vi "GPS -Nearest Points to Lat Lng.vi"(5 "Inputs":T1={" # Pts"=5, "PinDropLatDblClck"=0.0, "PinDropLngDblClck"=0.0, "AddrLat"=0.0, "AddrLng"=0.0, "tbVw"=enum."Position"}, 11 "error in (no error)":errorcluster) -> (15 "error out":errorcluster)   [LabVIEW 2019]
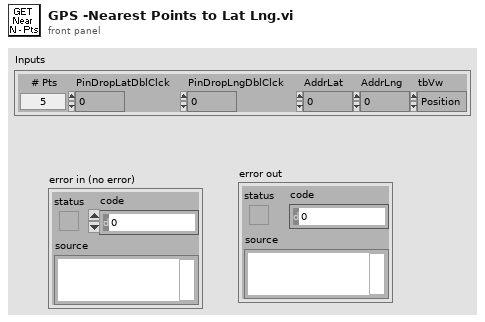
[diagram p1: front panel]
types:
  T1 = cluster{" # Pts":i32, "PinDropLatDblClck":dbl, "PinDropLngDblClck":dbl, "AddrLat":dbl, "AddrLng":dbl, "tbVw":enum32{"Position", "Pin Drop", "Addr", "Setup"}}
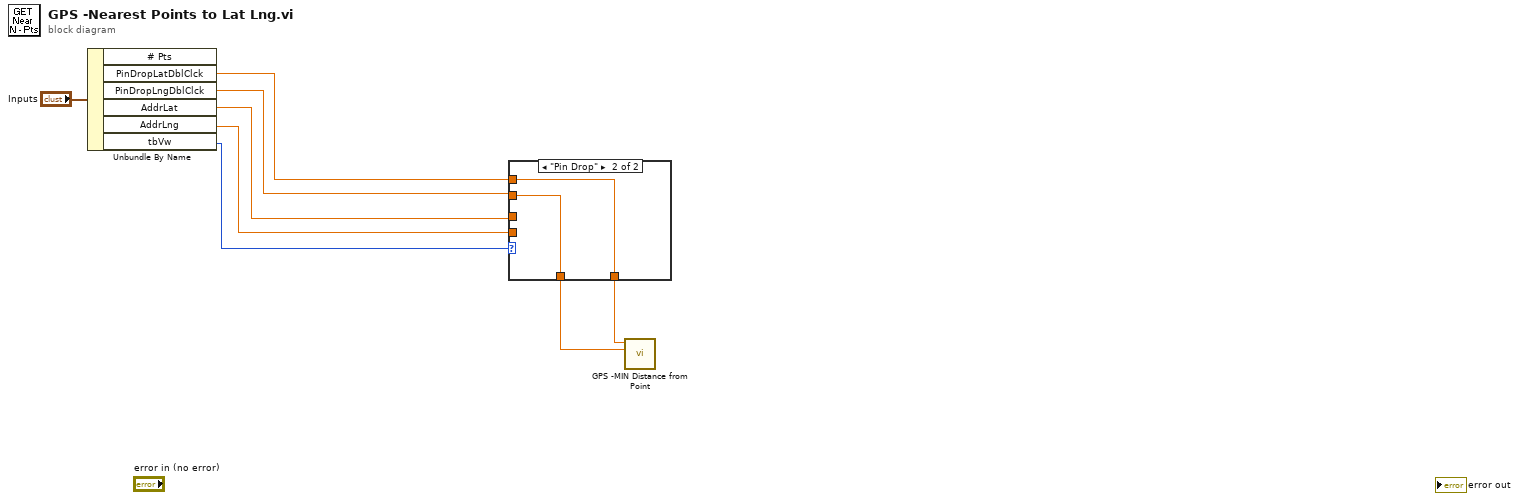
[diagram p0: block diagram]
diagram:
  n1 = Unbundle By Name("Inputs") -> ("PinDropLatDblClck"=w5:dbl, "PinDropLngDblClck"=w4:dbl, "AddrLat"=w3:dbl, "AddrLng"=w2:dbl, "tbVw"=w1:enum32{"Position", "Pin Drop", "Addr", "Setup"})  [unwired: 1 out]
  n2 = case shown="\"Pin Drop\"" w1 {
    tunnel: [w10 w12] -> w7
    tunnel: [w9 w11] -> w8
    tunnel: w2 -> [w10 _]
    tunnel: w3 -> [w9 _]
    tunnel: w4 -> [_ w12]
    tunnel: w5 -> [_ w11]
    frame "Addr", Default {
    }
    frame "Pin Drop" {
    }
  }
  n3 = call "GPS -MIN Distance from Point.vi"("POI-Lat"=w8, "POI-Lng"=w7) -> ()  [unwired: 16 in, 2 out]
